vi "group Sync Read Is Available.vi"(7 "data_length":u16, 9 "address":u16, 10 "id":u8, 11 "group_num":i32) -> (3 "function return":u8)   [LabVIEW 2016, in "dxl_x86_c.lvlib"]
doc: "WINDECLSPEC uint8_t groupSyncReadIsAvailable (int group_num, uint8_t id, uint16_t address, uint16_t data_length);"
uses:
  dxl_x86_c.lvlib
  dxl_x86_c.dll
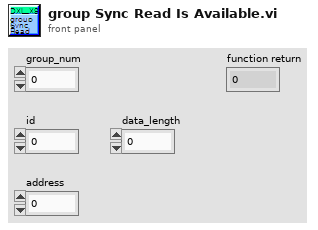
[diagram p1: front panel]
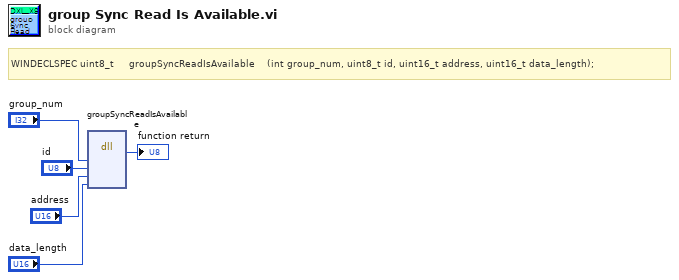
[diagram p0: block diagram]
diagram:
  # "WINDECLSPEC uint8_t     groupSyncReadIsAvailable    (int group_num, uint8_t id, uint16_t address, uint16_t data_length);"
  n1 = dll-call lib="C:/Users/Platform/Desktop/DynamixelSDK/labview/dxl_x86_c.lvlib/dxl_x86_c.*" fn="groupSyncReadIsAvailable"("group_num"="group_num", "id"="id", "address"="address", "data_length"="data_length") -> (→"function return":u8)  [unwired: 7 in, 2 out]
